vi "Stop Core.vi"(10 "final error code":i32, 11 "[MDI] Child in":refnum<class "[MDI] Child.lvclass">) -> (3 "[MDI] Child out":refnum<class "[MDI] Child.lvclass">)   [LabVIEW 2020, in "[MDI] Child.lvlib" / "[MDI] Child.lvclass"]
doc: "(<B>Filename</B>: Actor Framework.lvlib:Actor.lvclass:Stop Core.vi)\n\nDefines what the actor does before it stops. Use the <B>final error code</B> input to determine whether the actor shut down in response to an error.\n\nBy default, this method passes the Stop message along to all auto-stop nested actors. A descendant class may override this method to define additional behavior, such as shutting down any processes the actor initiated in its override of the Actor Core method."
uses:
  [MDI] Child.lvclass
  C:/Program Files (x86)/National Instruments/LabVIEW 2020/vi.lib/ActorFramework/Actor/Actor.lvclass
  <vilib>/ActorFramework/Actor/Actor.lvclass/Actor.ctl
  [MDI] Child.lvclass/[MDI] Child.ctl
  [MDI] Parent/[MDI] Parent Messages/Remove Child Msg/Remove Child Msg.lvclass/Remove Child Msg.ctl
  <vilib>/ActorFramework/Message Enqueuer/Message Enqueuer.lvclass/Message Enqueuer.ctl
  Accessor/Read Child Name.vi
  <vilib>/ActorFramework/Message Enqueuer/Enqueue.vi
  [MDI] Parent/[MDI] Parent Messages/Remove Child Msg/Remove Child Msg.lvclass
  C:/Program Files (x86)/National Instruments/LabVIEW 2020/vi.lib/ActorFramework/Message/Message.lvclass
  <vilib>/ActorFramework/Message Priority Queue/Priority Enqueue.vi
  <vilib>/ActorFramework/Actor/Actor.lvclass
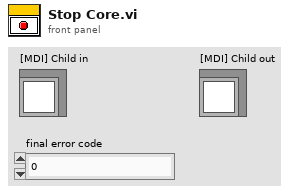
[diagram p1: front panel]
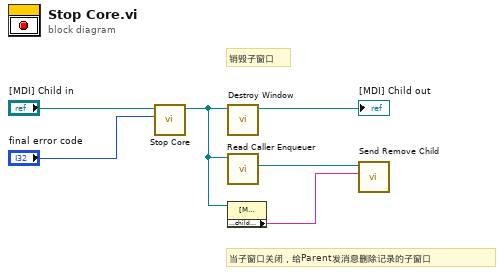
[diagram p0: block diagram]
diagram:
  # "销毁子窗口"
  # "当子窗口关闭，给Parent发消息删除记录的子窗口"
  n1 = call-parent "Stop Core.vi"("final error code"="final error code", "Actor in"="[MDI] Child in") -> ("Actor out"=w3:refnum<class "[MDI] Child.lvclass">)  [unwired: 9 in]
  n2 = call "Destroy Window.vi"("[MDI] Child in"=w3) -> ("[MDI] Child out"=→"[MDI] Child out":refnum<class "[MDI] Child.lvclass">)  [unwired: 9 in, 1 out]
  n3 = call <vilib>:"Read Caller Enqueuer.vi"("Actor"=w3) -> ("Caller Enqueuer"=w2:refnum<class "Message Enqueuer.lvclass">)  [unwired: 10 in]
  n4 = property class="[MDI] Child.lvclass"(reference=w3) -> ("Accessor:child name"=w1:string)  [unwired: 1 in, 2 out]
  n5 = call "Send Remove Child.vi"("child name"=w1, "Message Enqueuer"=w2) -> ()  [unwired: 8 in, 2 out]
